vi "InitialSMT.vi"(8 "error in (no error)":errorcluster, 11 "Programing Logic in":refnum<class "Programing Logic.lvclass">) -> (0 "error out":errorcluster, 2 "Reconnect":bool, 3 "Programing Logic out":refnum<class "Programing Logic.lvclass">)   [LabVIEW 2014, in "Programing Logic.lvclass"]
uses:
  Programing Logic.lvclass
  Programing Logic.lvclass/Programing Logic.ctl
panel:
  out "STM2":bool
  out "STM1":bool
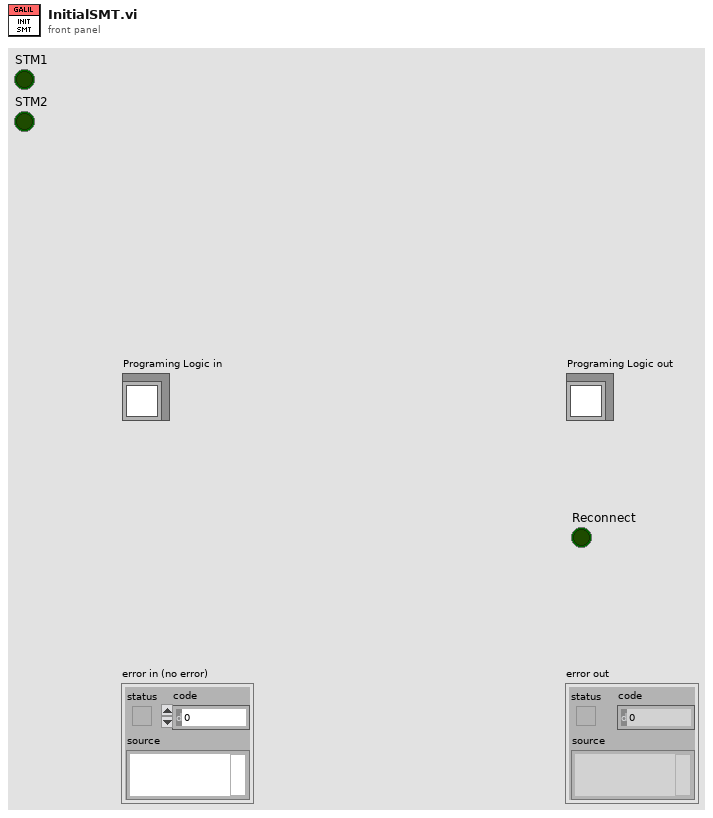
[diagram p1: front panel]
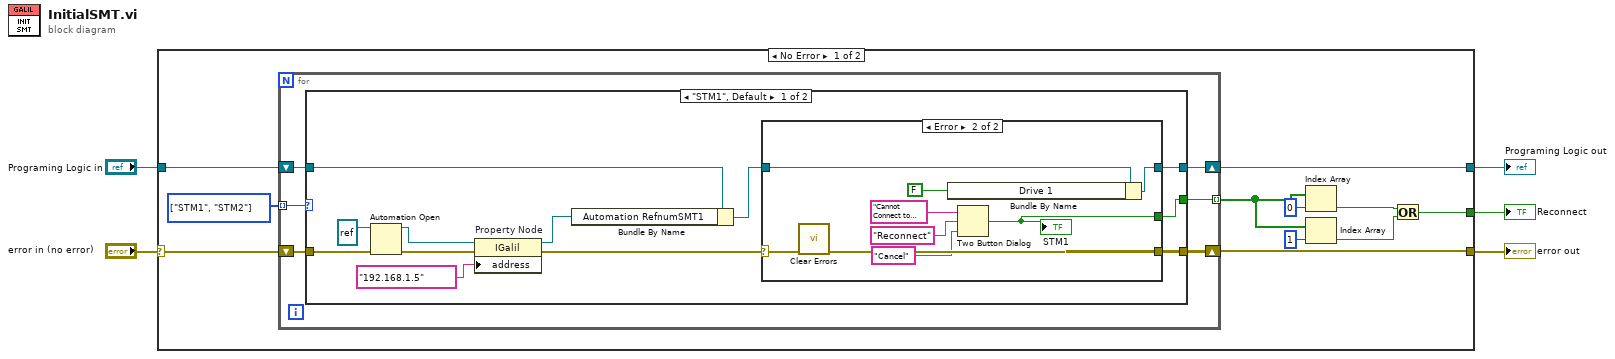
[diagram p0: block diagram]
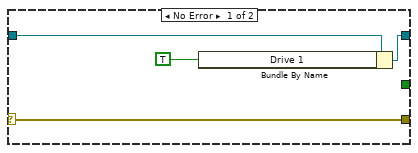
[diagram p2: hidden frame]
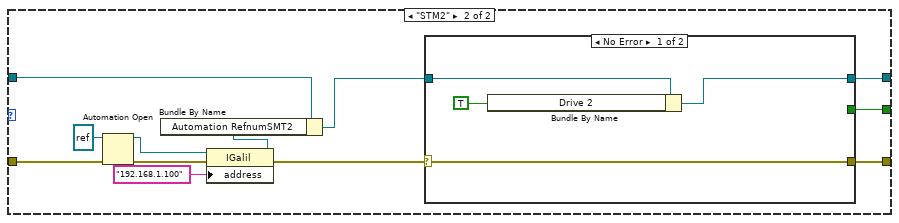
[diagram p3: hidden frame]
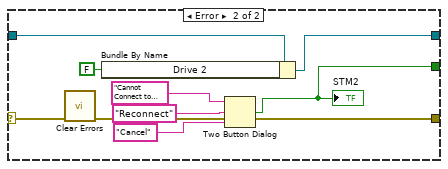
[diagram p4: hidden frame]
diagram:
  n1 = case shown="No Error" "error in (no error)" {
    selector: "error in (no error)" -> [w16 w74]
    tunnel: [w12 w74] -> w4
    tunnel: [w13 w73] -> w3
    tunnel: "Programing Logic in" -> [w15 w73]
    tunnel: [w11 _] -> w1
    frame No Error {
      w14 = enum16{"STM1", "STM2"}[] [enum."STM1", enum."STM2"] items=["STM1", "STM2"]
      n2 = for {
        shift-right: [w21] -> w12
        shift-left: w16 -> [w22]
        shift-right: [w19] -> w13
        shift-left: w15 -> [w20]
        tunnel: w14 -> [w18] mode=indexing
        tunnel: [w17] -> w7 mode=indexing
        n3 = case shown="\"STM1\", Default" w18 {
          tunnel: w22 -> [w33 w59]
          tunnel: [w24 w50] -> w21
          tunnel: w20 -> [w29 w55]
          tunnel: [w26 w51] -> w19
          tunnel: [w23 w48] -> w17
          frame "STM1", Default {
            n4 = Automation Open(error in (no error)=w33, Automation Refnum=refnum<k7> refnum ("Automation Refnum in")) -> (Automation Refnum=w32:refnum<k7>, error out=w31:errorcluster)  [unwired: 2 in]
            n5 = property on="Property Node" class="IGalil"(reference=w32, error in=w31, "address"="192.168.1.5") -> (reference out=w28:refnum<k7>, error out=w25:errorcluster)
            n6 = Bundle By Name(cluster=w29, "Automation RefnumSMT1"=w28) -> (w27:refnum<class "Programing Logic.lvclass">)
            n7 = case shown="Error" w25 {
              selector: w25 -> [w38 w45]
              tunnel: [w36 w43] -> w26
              tunnel: w27 -> [w37 w44]
              tunnel: [w38 w46] -> w24
              tunnel: [_ w39] -> w23
              frame No Error {
                n8 = Bundle By Name(cluster=w37, "Drive 1"=TRUE) -> (w36:refnum<class "Programing Logic.lvclass">)
              }
              frame Error {
                n9 = call <vilib>:"Clear Errors.vi"("error in (no error)"=w45) -> ("error out"=w46:errorcluster)  [unwired: 5 in, 1 out]
                n10 = Bundle By Name(cluster=w44, "Drive 1"=FALSE) -> (w43:refnum<class "Programing Logic.lvclass">)
                n11 = Two Button Dialog(message="Cannot Connect to   Drive 1 ", 1:"Cancel" ("F button name (\"Cancel\")"), 2:"Reconnect" ("button name (\"OK\")")) -> (T button?=w39:bool)
                "STM1" <- w39
              }
            }
          }
          frame "STM2" {
            n12 = Automation Open(error in (no error)=w59, Automation Refnum=refnum<k7> refnum) -> (Automation Refnum=w58:refnum<k7>, error out=w57:errorcluster)  [unwired: 2 in]
            n13 = property on="Property Node" class="IGalil"(reference=w58, error in=w57, "address"="192.168.1.100") -> (reference out=w54:refnum<k7>, error out=w49:errorcluster)
            n14 = Bundle By Name(cluster=w55, "Automation RefnumSMT2"=w54) -> (w52:refnum<class "Programing Logic.lvclass">)
            n15 = case shown="No Error" w49 {
              selector: w49 -> [w63 w70]
              tunnel: w52 -> [w61 w69]
              tunnel: [w60 w68] -> w51
              tunnel: [w63 w71] -> w50
              tunnel: [_ w64] -> w48
              frame No Error {
                n16 = Bundle By Name(cluster=w61, "Drive 2"=TRUE) -> (w60:refnum<class "Programing Logic.lvclass">)
              }
              frame Error {
                n17 = call <vilib>:"Clear Errors.vi"("error in (no error)"=w70) -> ("error out"=w71:errorcluster)  [unwired: 5 in, 1 out]
                n18 = Bundle By Name(cluster=w69, "Drive 2"=FALSE) -> (w68:refnum<class "Programing Logic.lvclass">)
                n19 = Two Button Dialog(message="Cannot Connect to   Drive 2 ", 1:"Cancel" ("F button name (\"Cancel\")"), 2:"Reconnect" ("button name (\"OK\")")) -> (T button?=w64:bool)
                "STM2" <- w64
              }
            }
          }
        }
      }
      n20 = Index Array(array=w7, index=0) -> (element=w9:bool)
      n21 = Index Array(array=w7, index=1) -> (element=w8:bool)
      n22 = Or(x=w9, y=w8) -> (x .or. y?=w11:bool)
    }
    frame Error {
    }
  }
  "error out" <- w4
  "Programing Logic out" <- w3
  "Reconnect" <- w1
